vi "cdaq_anal_write_dac_loop.vi"(8 "error in":errorcluster, 9 "fs [Hz]":dbl=50000.0 format="%#_13g", 10 "wave":dbl[](array[numeric]), 11 "cdaq session in":T1={"mclk [Hz]"=12800000.0, "DAC device"="", "ADC device"="", "DAC task"="", "ADC task"="", "adc idn"="", "dac idn"="", "fs [Hz]"=50000.0, "queue adc cmd"=refnum, "queue adc data"=refnum, "adc proc ref"=refnum}) -> (0 "error out":errorcluster, 2 "actual fs [Hz]":dbl, 3 "cdaq session out":T1={"mclk [Hz]"=12800000.0, "DAC device"="", "ADC device"="", "DAC task"="", "ADC task"="", "adc idn"="", "dac idn"="", "fs [Hz]"=50000.0, "queue adc cmd"=refnum, "queue adc data"=refnum, "adc proc ref"=refnum})   [LabVIEW 2020]
uses:
  cdaq_anal_session.ctl
  cdaq_anal_adc_command.ctl
  cdaq_anal_adc_data.ctl
  <vilib>/DAQmx/write.llb/DAQmx Write (Analog 1D DBL 1Chan NSamp).vi
  <vilib>/DAQmx/configure/timing.llb/DAQmx Timing (Sample Clock).vi
  <vilib>/DAQmx/miscellaneous.llb/DAQmx Fill In Error Info.vi
  <resource>/objmgr/daqmx.rc
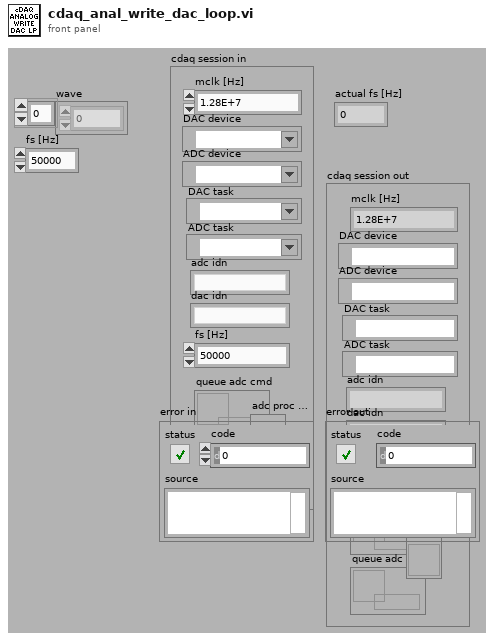
[diagram p1: front panel]
types:
  T1 = typedef "cdaq_anal_session.ctl" = cluster{"mclk [Hz]":dbl, "DAC device":tag, "ADC device":tag, "DAC task":refnum<k21>, "ADC task":refnum<k21>, "adc idn":string, "dac idn":string, "fs [Hz]":dbl, "queue adc cmd":refnum<queue>, "queue adc data":refnum<queue>, "adc proc ref":refnum<vi>}
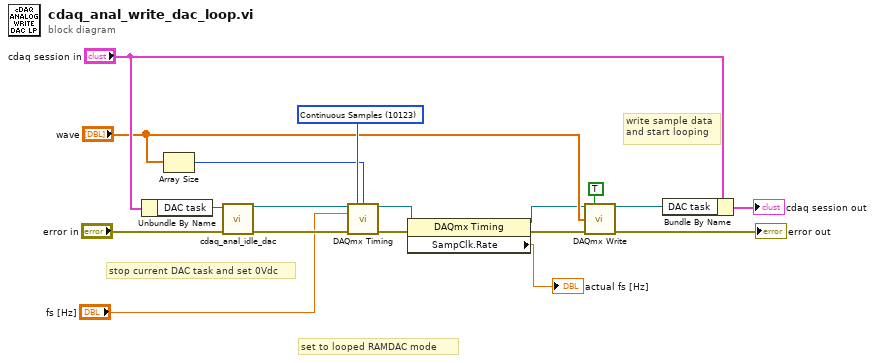
[diagram p0: block diagram]
diagram:
  w13 = 10123 items=["Finite Samples"=10178, "Continuous Samples"=10123, "Hardware Timed Single Point"=12522] ("sample mode")
  # "write sample data\nand start looping"
  # "set to looped RAMDAC mode"
  # "stop current DAC task and set 0Vdc"
  n1 = Unbundle By Name("cdaq session in") -> ("DAC task"=w18:refnum<k21>)
  n2 = Array Size(array="wave") -> (size(s)=w12:i32)
  n3 = call "cdaq_anal_idle_dac.vi"("error in"="error in", "task in"=w18) -> ("error out"=w14:errorcluster, "task out"=w11:refnum<k21>)  [unwired: 8 in]
  n4 = call-poly <vilib>:"DAQmx Timing.vi"("task/channels in"=w11, "sample mode"=w13, "samples per channel"=w12, "rate"="fs [Hz]", "error in"=w14) -> ("task out"=w4:refnum<k21>, "error out"=w5:errorcluster)  [unwired: 9 in]
  n5 = property class="DAQmx Timing"(reference=w4, error in=w5) -> (reference out=w2:refnum<k21>, error out=w3:errorcluster, "SampClk.Rate"=→"actual fs [Hz]":dbl)
  n6 = call-poly <vilib>:"DAQmx Write.vi"("task/channels in"=w2, "auto start"=TRUE, "data"="wave", "error in"=w3) -> ("task out"=w6:refnum<k21>, "error out"=→"error out":errorcluster)  [unwired: 9 in, 1 out]
  n7 = Bundle By Name(cluster="cdaq session in", "DAC task"=w6) -> (→"cdaq session out":T1)
